vi "DigitalOszi_PXIe-7962R.vi"() -> ()   [LabVIEW 2012]
uses:
  <vilib>/Platform/TimedLoop/XDataNode/timing_clust.ctl
  <vilib>/Platform/TimedLoop/XDataNode/nitl_modes.ctl
  <vilib>/Platform/TimedLoop/XDataNode/wakeup.ctl
  <vilib>/rvi/Emulation/niFpgaSctlEmulationRegisterWithScheduler.vi
  <vilib>/rvi/eio/common/nirviEmuTemplateMethod_errors.vi
  <vilib>/rvi/Emulation/niFpgaSctlEmulationScheduler.vi
  <vilib>/rvi/DataTransferAndStorage/Container/Common/niFpgaContainerGetUniqueNameForEmu.vi
  <vilib>/rvi/FIFO/Fifo_Resource/nirvififoEmulationSetSize.vi
  <vilib>/rvi/errors/niFpgaSetErrorForExecOnDevCompSimple.vi
  <vilib>/rvi/eio/common/nirviEmuReportErrorAndStop.vi
  <vilib>/rvi/Emulation/niFpgaSctlEmulationFifoFullMgr.vi
  <vilib>/rvi/Emulation/niFpgaSctlEmulationResourceMgr.vi
  <vilib>/rvi/interface/RandomDataEmulation/nirviRandomDataFPGAFIFO.vi
  <vilib>/rvi/interface/RandomDataEmulation/niFpgaRandomDataHandleErrors.vi
  <vilib>/Platform/TimedLoop/XDataNode/XDataNode.xnode
  <vilib>/eio/EIONode/EIONode.xnode
  <vilib>/rvi/DataTransferAndStorage/Container/XNode/niFpgaContainer.xnode
  <vilib>/rvi/FIFO/Fifo_Resource/nirvififoEmulationWrite.vi
  <vilib>/rvi/FIFO/Fifo_Resource/nirvififoEmulationRead.vi
  <vilib>/rvi/interface/RandomDataEmulation/nirviRandomDataFpgaReadWriteTemplate.vi
  <vilib>/Platform/TimedLoop/XDataNode/XDNodeRunTimeDep.lvlib
panel:
  out "Interloop FIFO overflow":bool
  in  "Onboard_Clock_Write_Data":u16 format="%b"
  in  "Onboard_Clock_Write":bool
  out "Onboard_Clock_Ready":bool
  out "ToHost overflow":bool
  out "Interloop Timed Out?":bool
  in  "Start Acq":bool
  in  "IO Module\\Acq_Reset":bool
  in  "Clock Source":u8(ring)=3 caption="Acq_IO_Clock_Source" items=["Tristate"=0, "Sync Clock (PXIe Only)"=2, "Adapter Module Onboard Clock"=3, "Strobe From Crosspoint Switch"=4, "Strobe Bypass"=5]
  in  "Xpoint_Switch_Write":bool
  out "Xpoint_Switch_Ready":bool
  in  "Commit":bool
  # "Configuration"
  # "Acquisition"
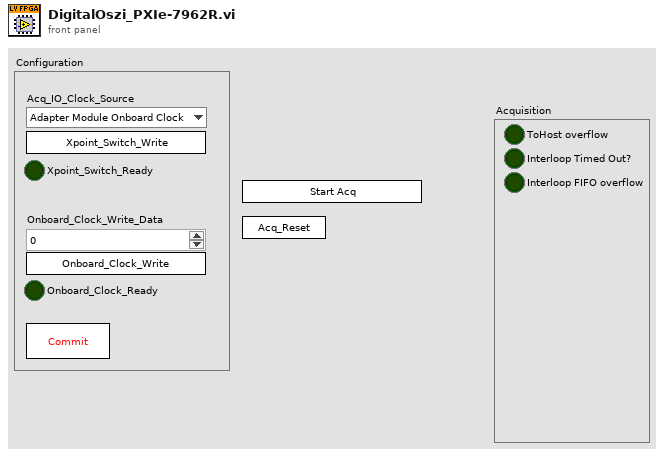
[diagram p1: front panel]
types:
  T1 = typedef "XDNodeRunTimeDep.lvlib/timing_clust.ctl" = cluster{"Expected End [f-1]":u64, "Actual End [f-1]":u64, "Finished Late? [f-1]":bool, "Expected End [i-1]":u64, "Actual End [i-1]":u64, "Finished Late? [i-1]":bool, "Expected Start [i]":u64, "Actual Start [i]":u64, "Expected Start [f]":u64, "Actual Start [f]":u64, "Source Name":string, "Structure Name":string, "Period":i64, "Deadline":i64, "Offset":i64, "Start":i64, "Priority":i32, "Timeout":i32, "Mode":T2, "Wakeup Reason":T3, "Error":errorcluster, "Source Type":string, "Secondary Source Type":string, "Global End Time":u64, "Global Start Time":u64, "Frame Duration":u64, "Iteration Duration":u64, "Assigned CPU":i32, "I/O Scan Engine Mode":u32}
  T2 = typedef "XDNodeRunTimeDep.lvlib/nitl_modes.ctl" = enum32{"No Change", "Process missed periods, maintain original phase", "Discard missed periods, maintain original phase", "Process missed periods, ignore original phase", "Discard missed periods, ignore original phase"}
  T3 = typedef "XDNodeRunTimeDep.lvlib/wakeup.ctl" = enum32{"Normal", "Aborted", "Asynchronous wakeup", "Timing source error", "Timed loop error", "Timeout"}
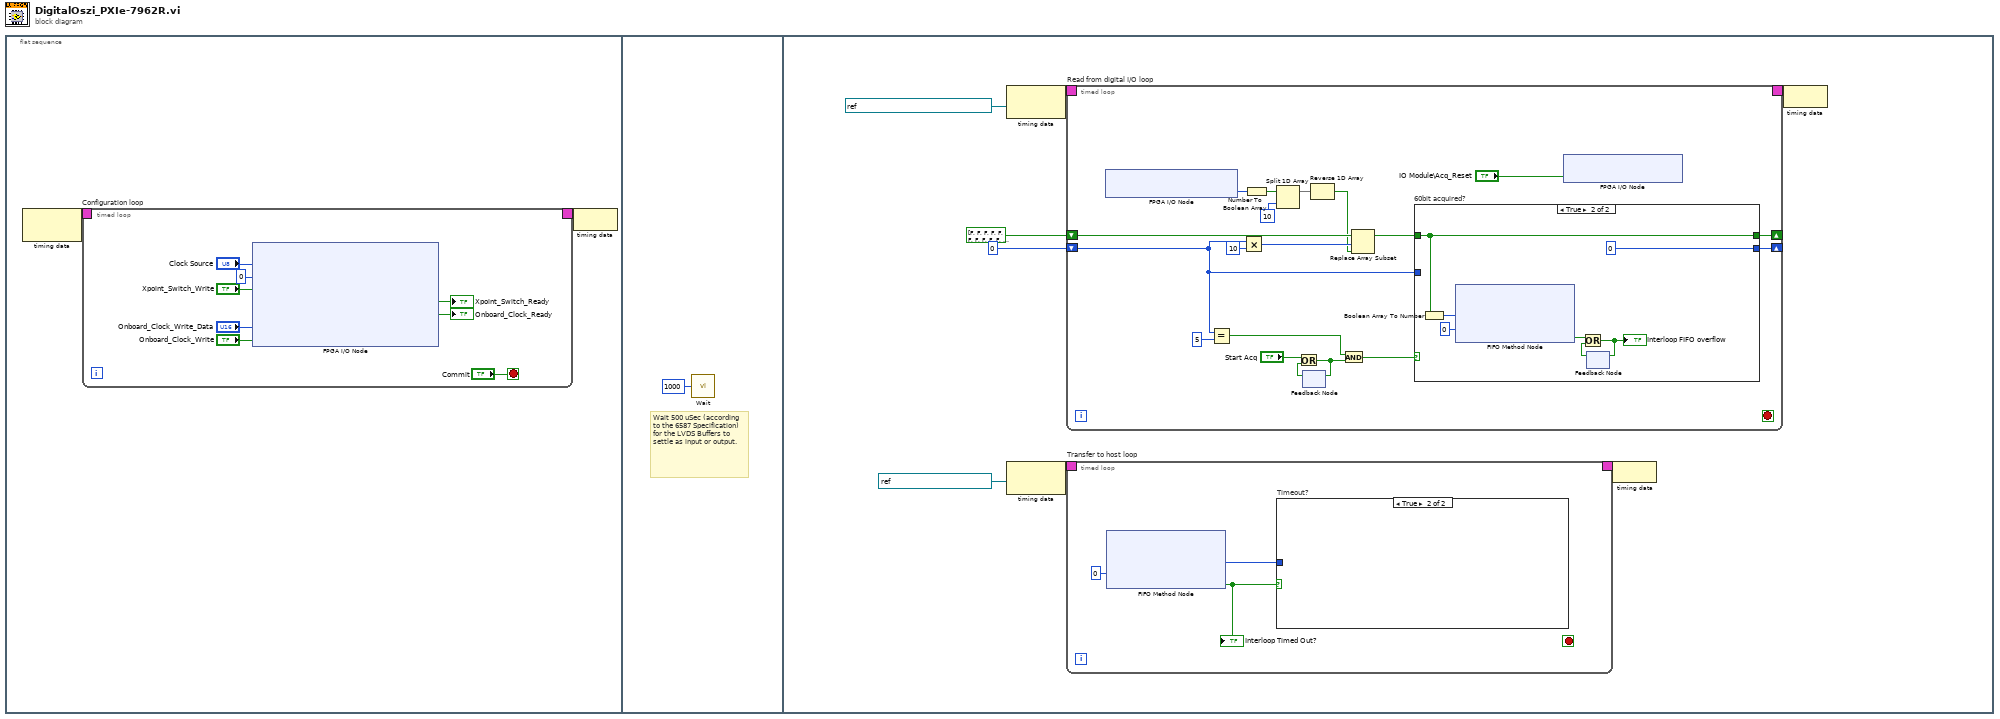
[diagram p0: block diagram]
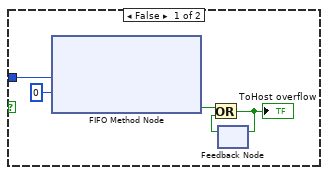
[diagram p2: hidden frame]
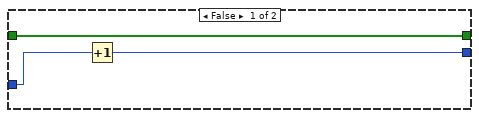
[diagram p3: hidden frame]
diagram:
  n1 = flat-sequence {
    frame #0 {
      n2 = node-c288() -> (w2:T1)  [unwired: 1 in]
      n3 = timed-loop "Configuration loop" {
        timing: w2 -> [_]
        timing-out: [_] -> w1
        stop <- "Commit" stop-if-true
        n4 = xnode "FPGA I/O Node"("IO Module\\Acq_IO_Clock_Source"="Clock Source", "IO Module\\LVDS_Data_Dir"=u16 0 ("IO Module\\LVDS_Data_Dir"), "IO Module\\Xpoint_Switch_Write"="Xpoint_Switch_Write", "IO Module\\Onboard_Clock_Write_Data"="Onboard_Clock_Write_Data", "IO Module\\Onboard_Clock_Write"="Onboard_Clock_Write") -> ("IO Module\\Xpoint_Switch_Ready"=→"Xpoint_Switch_Ready":bool, "IO Module\\Onboard_Clock_Ready"=→"Onboard_Clock_Ready":bool)  [unwired: 7 in, 7 out]
      }
      n5 = node-c288(w1) -> ()
    }
    frame #1 {
      # "Wait 500 uSec (according to the 6587 Specification) for the LVDS Buffers to settle as input or output."
      n6 = call "Wait"("Count(uSec)"=u32 1000) -> ()  [unwired: 1 out]
    }
    frame #2 {
      n7 = node-c288(refnum<k21> "IO Module\\Acq_Regional_Clock" ("Source Name")) -> (w23:T1)
      n8 = node-c288(refnum<k21> "40 MHz Onboard Clock" ("Source Name")) -> (w21:T1)
      n9 = timed-loop "Read from digital I/O loop" {
        timing: w23 -> [_]
        timing-out: [_] -> w22
        shift-right: [w40] -> _
        shift-left: 0 -> [w41]
        shift-right: [w42] -> _
        shift-left: bool[] [FALSE, FALSE, FALSE, FALSE, FALSE, FALSE, FALSE, FALSE, FALSE, FALSE, FALSE, FALSE, FALSE, FALSE, FALSE, FALSE, FALSE, FALSE, FALSE, FALSE, FALSE, FALSE, FALSE, FALSE, FALSE, FALSE, FALSE, FALSE, FALSE, FALSE, FALSE, FALSE, FALSE, FALSE, FALSE, FALSE, FALSE, FALSE, FALSE, FALSE, FALSE, FALSE, FALSE, FALSE, FALSE, FALSE, FALSE, FALSE, FALSE, FALSE, FALSE, FALSE, FALSE, FALSE, FALSE, FALSE, FALSE, FALSE, FALSE, FALSE, FALSE, FALSE, FALSE, FALSE] ("Boolean array") -> [w44]
        stop <- _ stop-if-true
        n10 = xnode "FPGA I/O Node"() -> ("IO Module\\LVDS_Ch0_Rd"=w53:u16)  [unwired: 1 in, 1 out]
        n11 = Equal?(x=w41, y=5) -> (x = y?=w47:bool)
        n12 = Multiply(x=w41, y=10) -> (x*y=w45:i32)
        n13 = Number To Boolean Array(number=w53) -> (Boolean array=w52:bool[])
        n14 = Split 1D Array(array=w52, index=10) -> (first subarray=w39:bool[])  [unwired: 1 out]
        n15 = feedback #1() -> (w54:bool)  [unwired: 1 in]
        n16 = Or(x="Start Acq", y=w54) -> (x .or. y?=w50:bool)
        n17 = feedback-in #1(w50) -> ()
        n18 = Reverse 1D Array(array=w39) -> (reversed array=w38:bool[])
        n19 = And(x=w47, y=w50) -> (x .and. y?=w49:bool)
        n20 = Replace Array Subset(array=w44, new element=w38, index=w45) -> (w43:bool[])
        n21 = case "60bit acquired?" shown="True" w49 {
          tunnel: [w59 w63] -> w42
          tunnel: w43 -> [w59 w63]
          tunnel: [w58 0] -> w40
          tunnel: w41 -> [w57 _]
          frame False {
            n22 = Increment(x=w57) -> (x+1=w58:i32)
          }
          frame True {
            n23 = Boolean Array To Number(Boolean array=w63) -> (number=w64:u64)
            n24 = xnode ("FIFO Method Node")("Element"=w64, "Timeout"=0) -> ("Timed Out?"=w62:bool)  [unwired: 1 in, 1 out]
            n25 = feedback #2() -> (w60:bool)  [unwired: 1 in]
            n26 = Or(x=w62, y=w60) -> (x .or. y?=w61:bool)
            "Interloop FIFO overflow" <- w61
            n27 = feedback-in #2(w61) -> ()
          }
        }
        n28 = xnode "FPGA I/O Node"("IO Module\\Acq_Reset"="IO Module\\Acq_Reset") -> ()  [unwired: 1 in, 1 out]
      }
      n29 = timed-loop "Transfer to host loop" {
        timing: w21 -> [_]
        timing-out: [_] -> w20
        stop <- _ stop-if-true
        n30 = xnode ("FIFO Method Node")("Timeout"=0) -> ("Element"=w26:u64, "Timed Out?"=w24:bool)  [unwired: 1 in, 1 out]
        "Interloop Timed Out?" <- w24
        n31 = case "Timeout?" shown="True" w24 {
          tunnel: w26 -> [w31 _]
          frame False {
            n32 = xnode ("FIFO Method Node")("Element"=w31, "Timeout"=0) -> ("Timed Out?"=w29:bool)  [unwired: 1 in, 1 out]
            n33 = feedback #3() -> (w28:bool)  [unwired: 1 in]
            n34 = Or(x=w29, y=w28) -> (x .or. y?=w27:bool)
            "ToHost overflow" <- w27
            n35 = feedback-in #3(w27) -> ()
          }
          frame True {
          }
        }
      }
      n36 = node-c288(w20) -> ()
      n37 = node-c288(w22) -> ()
    }
  }
